vi "GetText.vi"(8 "error in":errorcluster, 11 "node in":refnum<class "LabVIEW Build Node.lvclass">) -> (0 "error out":errorcluster, 1 "additional text":string, 2 "text":string, 3 "node out":refnum<class "LabVIEW Build Node.lvclass">, 4 "glyph":string)   [LabVIEW 2014, in "LabVIEW Build Node.lvclass"]
doc: "Returns the text representation of the node used for the tree control."
uses:
  LabVIEW Build Node.lvclass
  LabVIEW Build Node.lvclass/LabVIEW Build Node.ctl
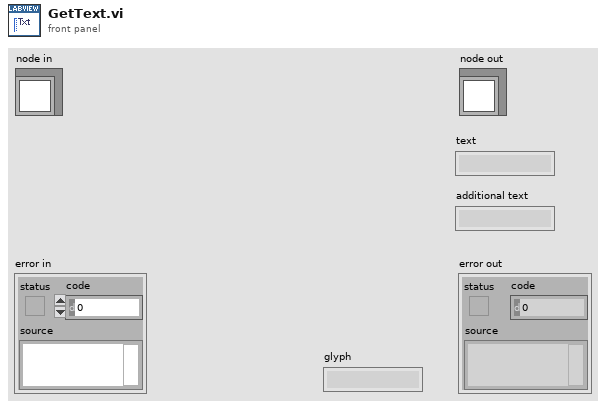
[diagram p1: front panel]
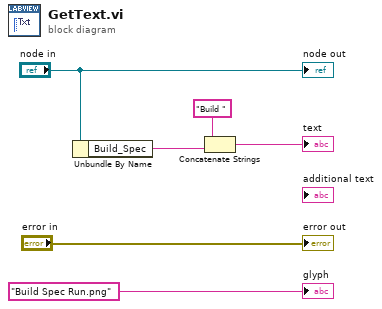
[diagram p0: block diagram]
diagram:
  n1 = Unbundle By Name("node in") -> ("Build_Spec"=w3:string)
  n2 = Concatenate Strings("Build " ("string"), w3) -> (→"text":string)
  "error out" <- "error in"
  "node out" <- "node in"
  "glyph" <- "Build Spec Run.png" ("glyph")
